vi "H5get_libversion.vi"(6 "error in (no error)":errorcluster) -> (0 "error out":errorcluster, 1 "Minor Version":u32, 2 "Major Version":u32, 3 "Version String":string, 4 "Release Number":u32)   [LabVIEW 2017]
doc: "Returns the HDF library release number."
uses:
  <vilib>/UPVI/lvhdf5/hdf5.dll
panel:
  # "LVHDF5 Toolkit\nCopyright (c) 2005-2013 by Jason D. Sommerville\nCopyright (c) 2014 by UPVI, LLC.\n\nThis use and distribution of this file is governed by the terms found in \nLICENSE.txt distributed with this toolkit and installed at\n <user.lib>\\_lvhdf5\\LICENSE.txt"
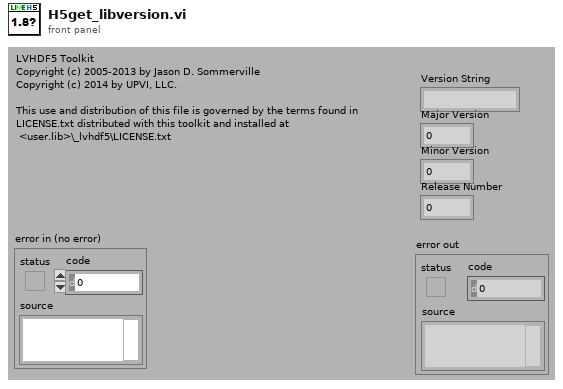
[diagram p1: front panel]
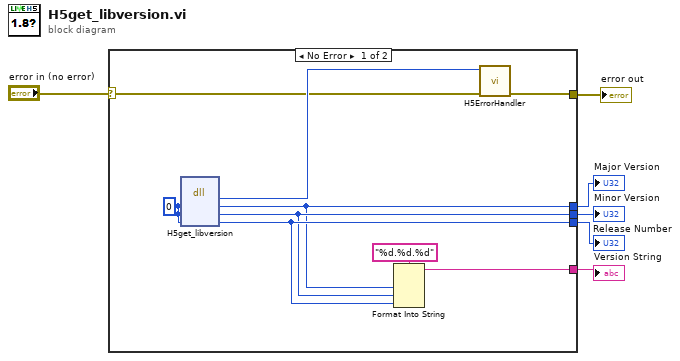
[diagram p0: block diagram]
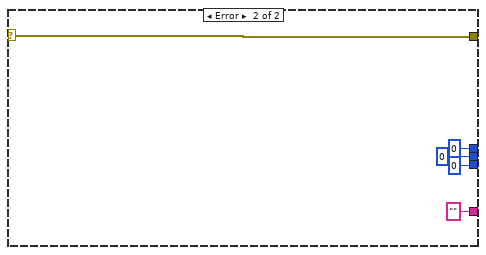
[diagram p2: hidden frame]
diagram:
  n1 = case shown="No Error" "error in (no error)" {
    selector: "error in (no error)" -> [w8 w20]
    tunnel: [w13 u32 0 ("relnum")] -> w1
    tunnel: [w12 u32 0 ("minnum")] -> w2
    tunnel: [w11 u32 0 ("majnum")] -> w3
    tunnel: [w10 ""] -> w4
    tunnel: [w7 w20] -> w5
    frame No Error {
      w15 = u32 0 ("majnum")
      n2 = dll-call lib="C:/Program Files/National Instruments/LabVIEW 2017/vi.lib/UPVI/lvhdf5/hdf5.dll" fn="H5get_libversion"("majnum"=w15, "minnum"=w15, "relnum"=w15) -> (w9:i32, "majnum"=w11:u32, "minnum"=w12:u32, "relnum"=w13:u32)  [unwired: 3 in, 2 out]
      n3 = Format Into String(format string="%d.%d.%d", w11, w12, w13) -> (resulting string=w10:string)  [unwired: 2 in, 1 out]
      n4 = call <vilib>:"H5ErrorHandler.vi"("error in (no error)"=w8, "herr_t"=w9) -> ("error out"=w7:errorcluster)  [unwired: 3 in, 4 out]
    }
    frame Error {
    }
  }
  "error out" <- w5
  "Version String" <- w4
  "Major Version" <- w3
  "Minor Version" <- w2
  "Release Number" <- w1
